vi "SEA_9811_RT_FIFO_processor.vi"(8 "error in (no error)":errorcluster, 10 "9811 Data in":u64[](array[numeric]), 11 "SEA9811_RT_data in":T1) -> (0 "error out":errorcluster, 3 "SEA9811_RT_data out":T1)   [LabVIEW 2012]
doc: "processes elements from FPGA and puts ARINC word and timestamp into DBL array"
uses:
  Typdefs/SEA9811_RT_data_cluster.ctl
  <userlib>/_FPGA Interface Advanced Tools/FPGA Interface Base/FPGA Interface Base.lvclass
  Typdefs/FPGA ref.ctl
  Typdefs/channel.ctl
  Typdefs/received word.ctl
  Typdefs/SEA9811_FPGA_FP_Addresses.ctl
  <userlib>/FPGA Timekeeper 1.1b0/FPGA Timekeeper.lvlib
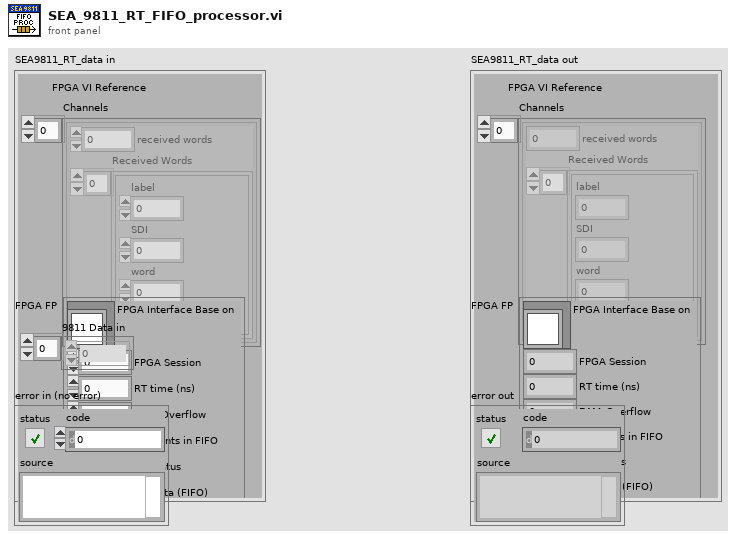
[diagram p1: front panel]
types:
  T1 = typedef "SEA9811_RT_data_cluster.ctl" = cluster{"FPGA VI Reference":T2, "Channels":T3[], "FPGA FP":T5}
  T2 = typedef "FPGA ref.ctl" = refnum<k20>
  T3 = typedef "channel.ctl" = cluster{"received words":u32, "Received Words":T4[]}
  T4 = typedef "received word.ctl" = cluster{"label":u8, "SDI":u8, "word":u32, "timestamp":dbl}
  T5 = typedef "SEA9811_FPGA_FP_Addresses.ctl" = cluster{"FPGA Interface Base on":refnum<class "FPGA Interface Base.lvclass">, "FPGA Session":u32, "RT time (ns)":u32, "DMA Overflow":u32, "Elements in FIFO":u32, "Rx Status":u32, "Rx Data (FIFO)":u32}
  T6 = typedef "ARINC word cluster.ctl" = cluster{"ARINC word":T7, "Label":u8, "SDI":u8, "Data":u32, "Parity":bool, "timestamp (DBL)":dbl}
  T7 = typedef "ARINC word.ctl" = u32
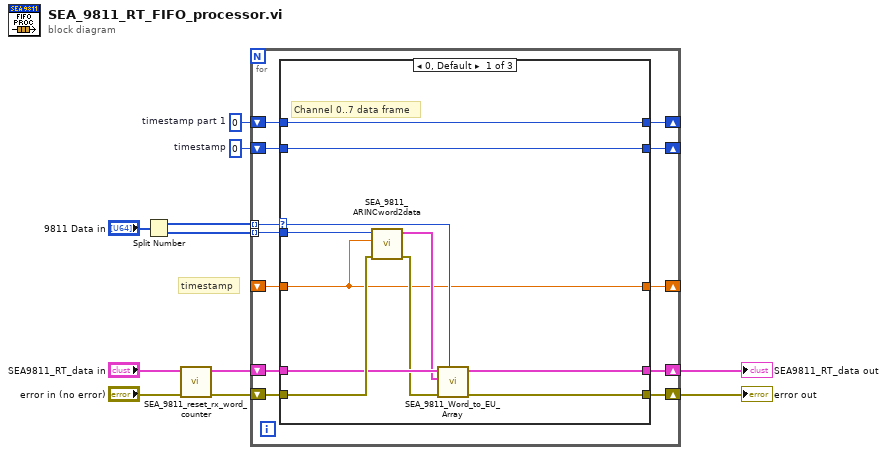
[diagram p0: block diagram]
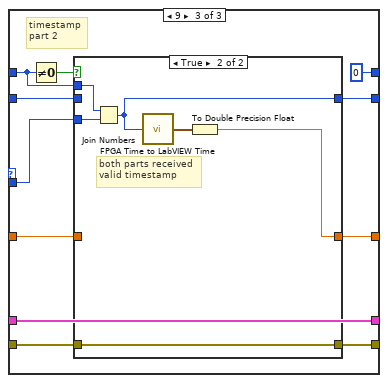
[diagram p3: hidden frame]
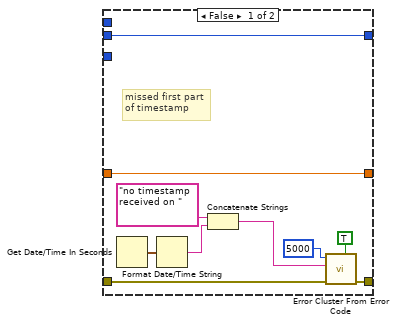
[diagram p4: hidden frame]
diagram:
  w7 = u32 0  # timestamp part 1
  w9 = u32 0  # timestamp
  # "timestamp"
  n1 = Split Number(x="9811 Data in") -> (hi(x)=w11:u32[], lo(x)=w10:u32[])
  n2 = call "SEA_9811_reset_rx_word_counter.vi"("error in (no error)"="error in (no error)", "SEA9811_RT_data in"="SEA9811_RT_data in") -> ("error out"=w1:errorcluster, "SEA9811_RT_data out"=w3:T1)  [unwired: 8 in]
  n3 = for {
    tunnel: w11 -> [w23] mode=indexing
    tunnel: w10 -> [w20] mode=indexing
    shift-right: [w22] -> _
    shift-left: w9 -> [w21]
    shift-right: [w19] -> _
    shift-left: w7 -> [w18]
    shift-right: [w16] -> w6
    shift-left: w1 -> [w17]
    shift-right: [w15] -> _
    shift-left: _ -> [w14]
    shift-right: [w12] -> w5
    shift-left: w3 -> [w13]
    n4 = case shown="0, Default" w23 {
      selector: w23 -> [w30 _ _]
      tunnel: [w34 w38 w45] -> w22
      tunnel: w21 -> [w34 w38 w46]
      tunnel: w20 -> [w25 w39 w47]
      tunnel: [w33 w39 u32 0] -> w19
      tunnel: w18 -> [w33 _ w48]
      tunnel: w17 -> [w32 w36 w44]
      tunnel: [w27 w36 w43] -> w16
      tunnel: [w24 w37 w42] -> w15
      tunnel: w14 -> [w24 w37 w41]
      tunnel: w13 -> [w31 w35 w40]
      tunnel: [w26 w35 w40] -> w12
      frame 0, Default {
        # "Channel 0..7 data frame"
        n5 = call "SEA_9811_ARINCword2data.vi"("error in (no error)"=w32, "timestamp (DBL) in"=w24, "ARINC word in"=w25) -> ("error out"=w28:errorcluster, "ARINC word out"=w29:T6)  [unwired: 7 in]
        n6 = call "SEA_9811_Word_to_EU_Array.vi"("Channel"=w30, "error in (no error)"=w28, "ARINC word in"=w29, "SEA9811_RT_data in"=w31) -> ("error out"=w27:errorcluster, "SEA9811_RT_data out"=w26:T1)  [unwired: 6 in]
      }
      frame 8 {
        # "timestamp\npart 1"
      }
      frame 9 {
        # "timestamp\npart 2"
        n7 = Not Equal To 0?(x=w48) -> (x != 0?=w49:bool)
        n8 = case shown="True" w49 {
          tunnel: w48 -> [_ w66]
          tunnel: w47 -> [_ w65]
          tunnel: w46 -> [w60 _]
          tunnel: [w60 w63] -> w45
          tunnel: w44 -> [w57 w64]
          tunnel: [w56 w64] -> w43
          tunnel: [w51 w61] -> w42
          tunnel: w41 -> [w51 _]
          frame False {
            # "missed first part\nof timestamp"
            n9 = Get Date/Time In Seconds() -> (seconds since 1Jan1904=w55:timestamp)
            n10 = Format Date/Time String(seconds (now)=w55) -> (date/time string=w53:string)  [unwired: 2 in]
            n11 = Concatenate Strings("no timestamp received on " ("string"), w53) -> (w52:string)
            n12 = call <vilib>:"Error Cluster From Error Code.vi"("is warning? (False)"=TRUE, "error in (no error)"=w57, "error message (\"\")"=w52, "error code (0)"=5000) -> ("error out"=w56:errorcluster)  [unwired: 5 in]
          }
          frame True {
            # "both parts received\nvalid timestamp"
            n13 = Join Numbers(hi=w66, lo=w65) -> ((hi.lo)=w63:u64)
            n14 = call <userlib>:"FPGA Time to LabVIEW Time.vi"("FPGA time (ns)"=w63) -> ("LabVIEW time"=w62:timestamp)
            n15 = To Double Precision Float(number=w62) -> (double precision float=w61:dbl)
          }
        }
      }
    }
  }
  "SEA9811_RT_data out" <- w5
  "error out" <- w6
